vi "N-216 Contol.vi"(0 "N-216 Notifier":refnum<notifier>, 5 "Stage Action":T1={"Action"=enum."Get Position", "Axis"=[], "Setpoint"=[], "Velocity"=0.5, "Cmd Recvd?"=FALSE, "Position"=[], "Status"=enum."Error", "Misc"=variant} {"Velocity" min=0.0 max=1.0 step=0.01}, 11 "VISA In":refnum<visa-resource-name>, 13 "Axis Name":string) -> (4 "N-216 Notifier (Dup)":refnum<notifier>)   [LabVIEW 2016]
uses:
  Stages Controls/Stage Notifier Element.ctl
  Stages Controls/Stage Actions.ctl
  Stages Controls/Stage Status.ctl
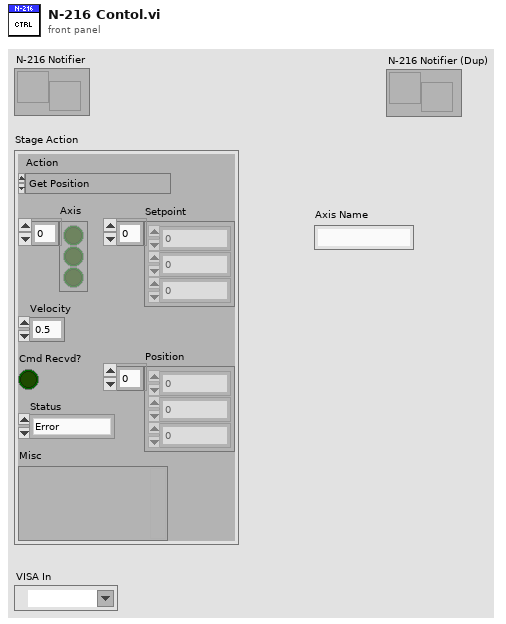
[diagram p1: front panel]
types:
  T1 = typedef "Stage Notifier Element.ctl" = cluster{"Action":T2, "Axis":bool[], "Setpoint":dbl[], "Velocity":dbl, "Cmd Recvd?":bool, "Position":dbl[], "Status":T3, "Misc":variant}
  T2 = typedef "Stage Actions.ctl" = enum16{"Get Position", "MVR", "MOVE", "HALT", "ONTARGET", "ERROR", "REFERENCE", "INIT", "VELOCITY", "STATUS", "EXIT", "HOME", "ZEROPOS", "NANOPOS", "ANALOG", "QUIT"}
  T3 = typedef "Stage Status.ctl" = enum16{"Error", "Abort", "Busy", "On Target"}
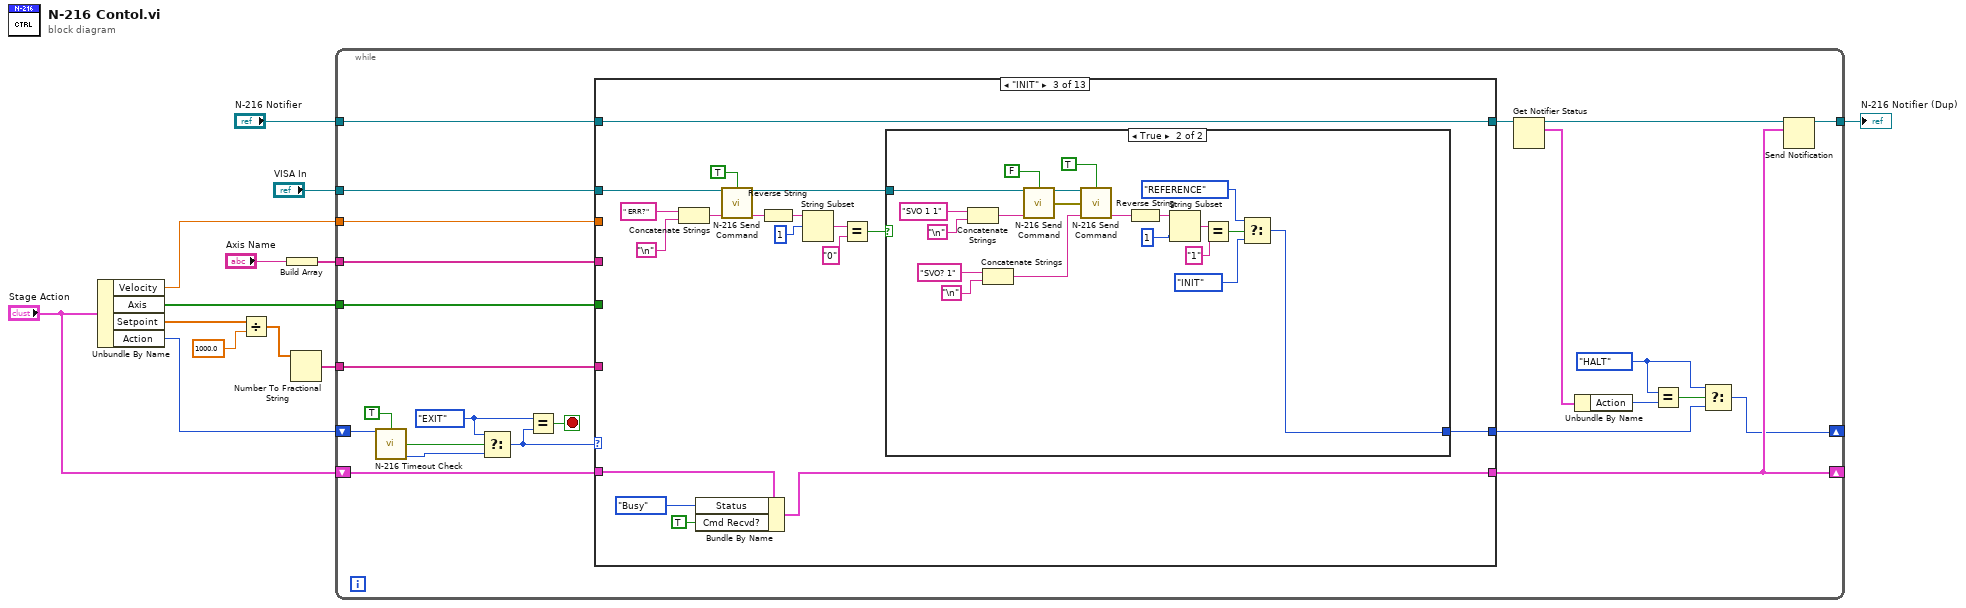
[diagram p0: block diagram]
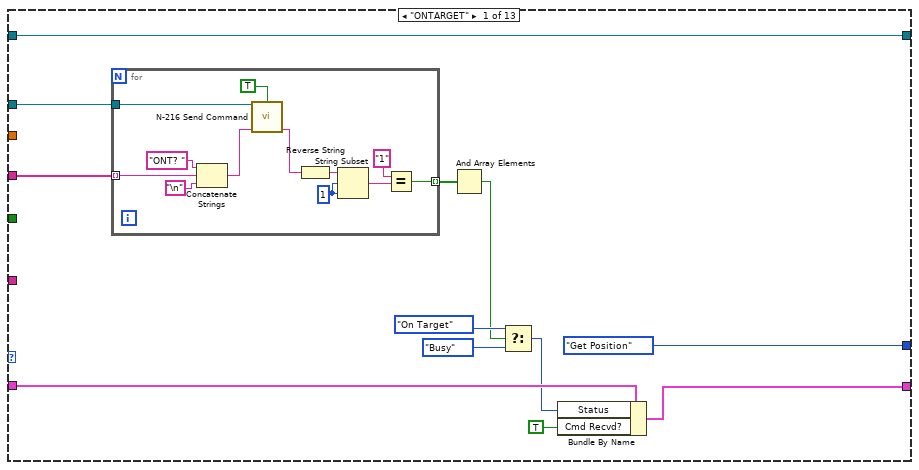
[diagram p2: hidden frame]
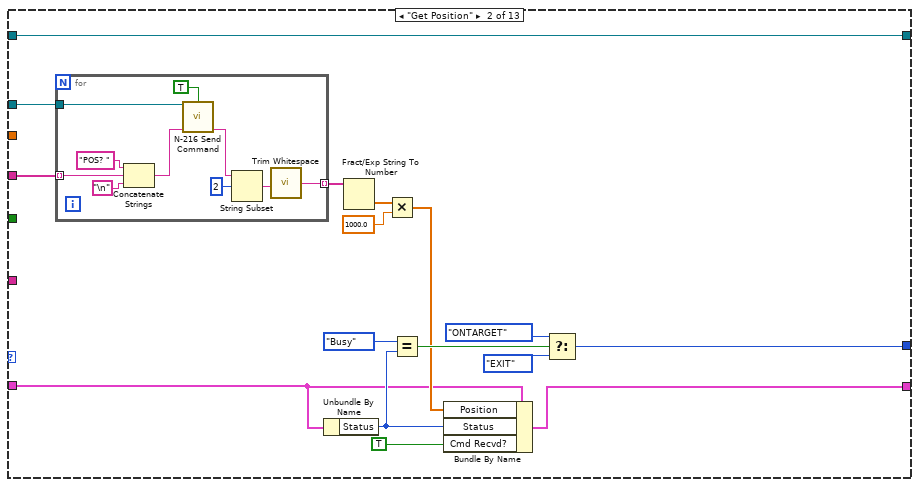
[diagram p3: hidden frame]
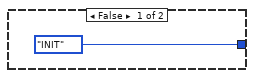
[diagram p4: hidden frame]
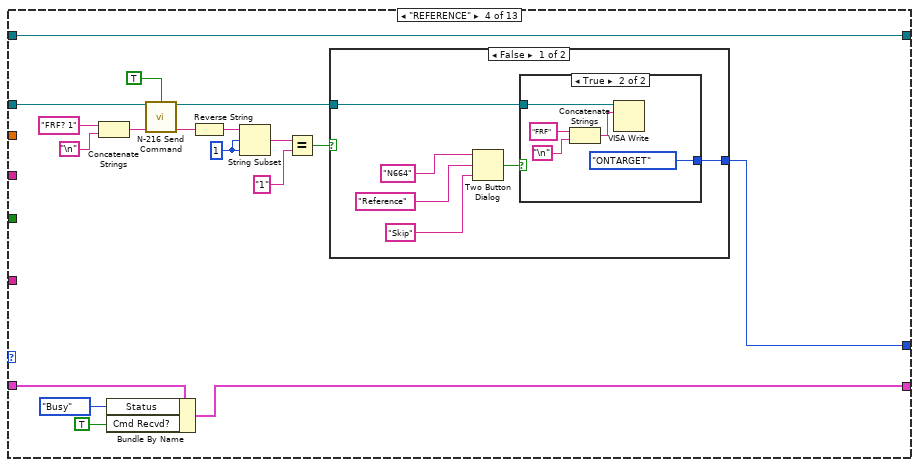
[diagram p5: hidden frame]
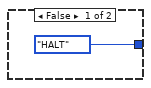
[diagram p6: hidden frame]
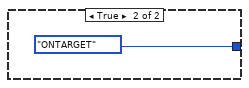
[diagram p7: hidden frame]
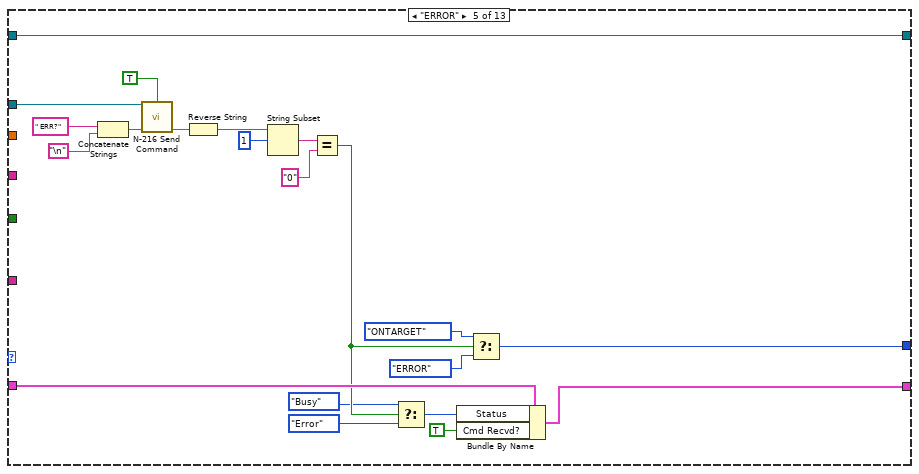
[diagram p8: hidden frame]
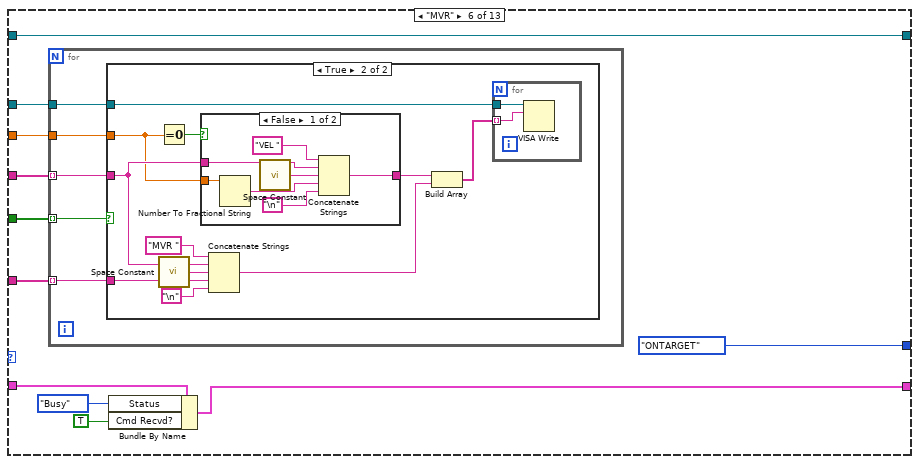
[diagram p9: hidden frame]
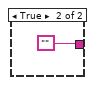
[diagram p11: hidden frame]
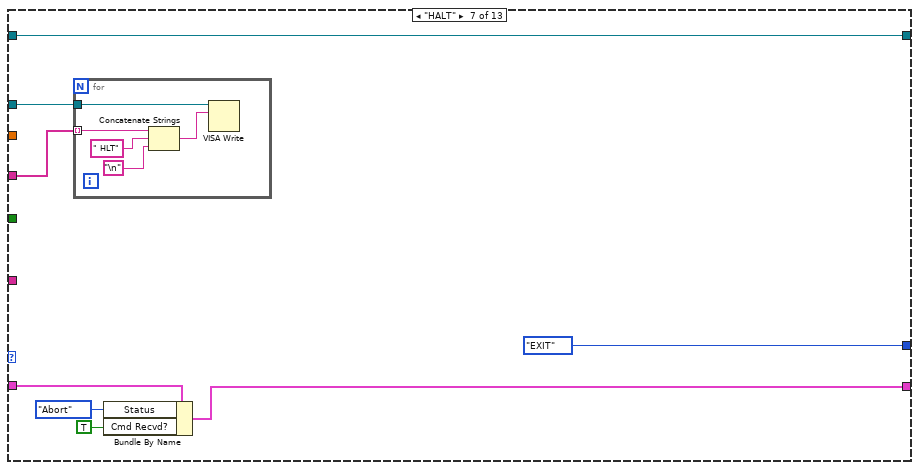
[diagram p12: hidden frame]
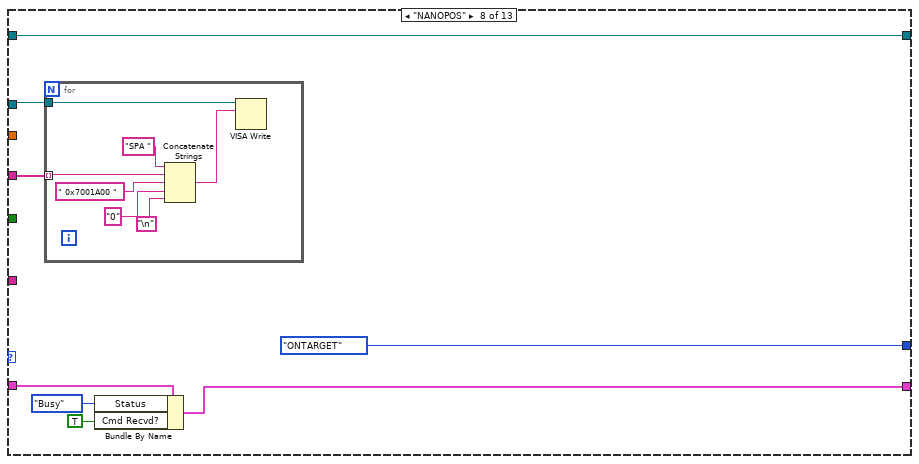
[diagram p13: hidden frame]
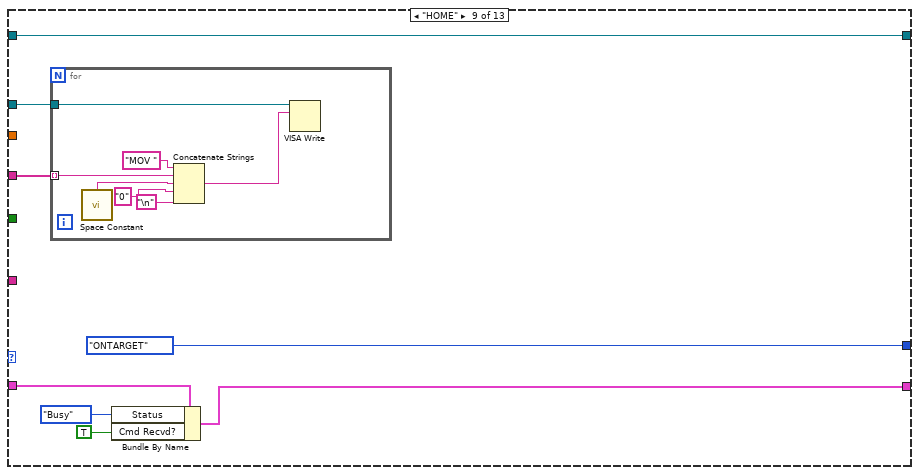
[diagram p14: hidden frame]
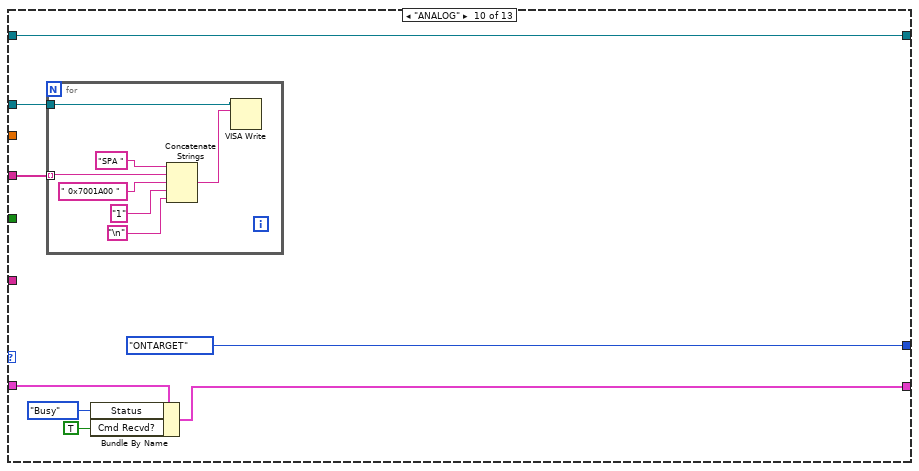
[diagram p15: hidden frame]
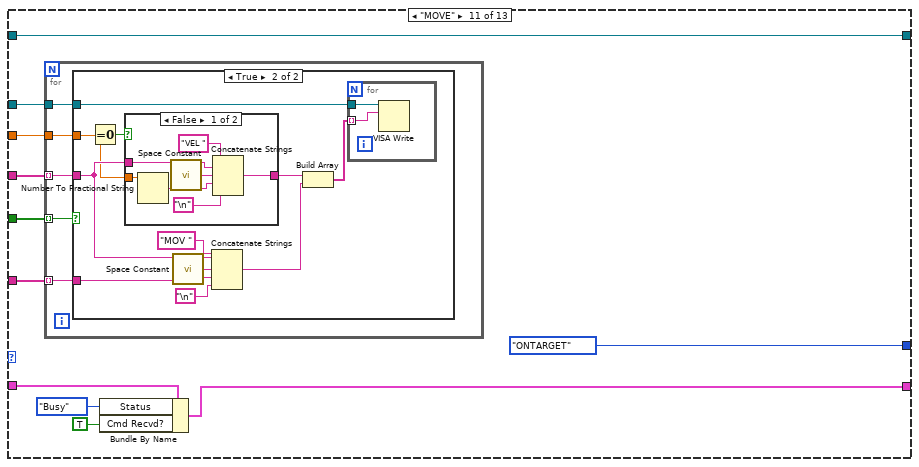
[diagram p16: hidden frame]
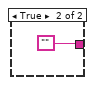
[diagram p18: hidden frame]
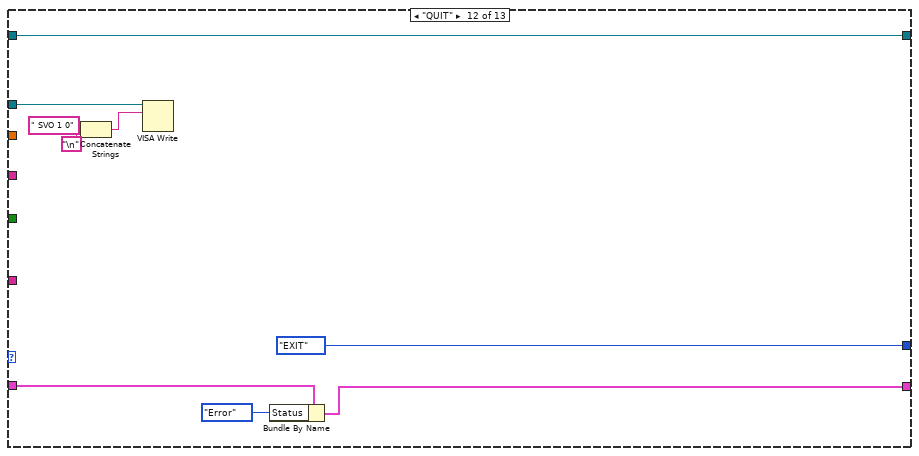
[diagram p19: hidden frame]
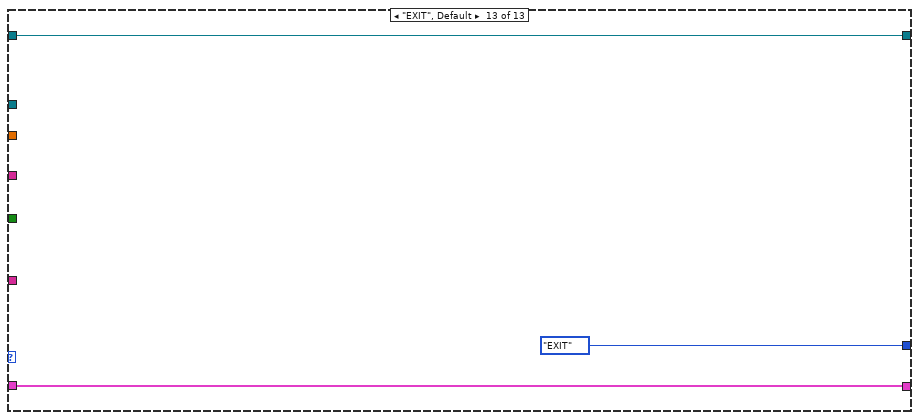
[diagram p20: hidden frame]
diagram:
  n1 = Unbundle By Name("Stage Action") -> ("Velocity"=w12:dbl, "Axis"=w11:bool[], "Setpoint"=w10:dbl[], "Action"=w9:T2)
  n2 = Divide(x=w10, y=1000.0) -> (x/y=w8:dbl[])
  n3 = Build Array("Axis Name") -> (w1:string[])
  n4 = Number To Fractional String(number=w8) -> (F-format string=w13:string[])  [unwired: 3 in]
  n5 = while {
    tunnel: w1 -> [w37]
    shift-right: [w16] -> _
    shift-left: w9 -> [w29]
    tunnel: w11 -> [w35]
    tunnel: w12 -> [w34]
    tunnel: w13 -> [w36]
    shift-right: [w31] -> _
    shift-left: "Stage Action" -> [w33]
    tunnel: "N-216 Notifier" -> [w23]
    tunnel: "VISA In" -> [w15]
    tunnel: [w14] -> w3
    stop <- w24 stop-if-true
    w19 = Stage_Actions."HALT" ("Action")
    w28 = Stage_Actions."EXIT" ("t")
    n6 = call "N-216 Timeout Check.vi"("Action"=w29, "User Input?"=TRUE) -> ("Timeout?"=w27:bool, "Action (Dup)"=w26:T2)  [unwired: 12 in]
    n7 = Select(t=w28, s=w27, f=w26) -> (s? t:f=w25:T2)
    n8 = Equal?(x=w28, y=w25) -> (x = y?=w24:bool)
    n9 = case shown="\"INIT\"" w25 {
      tunnel: w37 -> [w49 w77 _ _ _ w189 w223 w236 w251 w266 w284 _ _]
      tunnel: w15 -> [w38 w64 w93 w131 w161 w181 w217 w230 w245 w260 w274 w312 _]
      tunnel: w36 -> [_ _ _ _ _ w188 _ _ _ _ w283 _ _]
      tunnel: w35 -> [_ _ _ _ _ w187 _ _ _ _ w282 _ _]
      tunnel: w34 -> [_ _ _ _ _ w186 _ _ _ _ w281 _ _]
      tunnel: [Stage_Actions."Get Position" ("Action") w75 w105 w140 w173 Stage_Actions."ONTARGET" ("Action") Stage_Actions."EXIT" ("Action") Stage_Actions."ONTARGET" ("Action") Stage_Actions."ONTARGET" ("Action") Stage_Actions."ONTARGET" ("Action") Stage_Actions."ONTARGET" ("Action") Stage_Actions."EXIT" ("Action") Stage_Actions."EXIT" ("Action")] -> w32
      tunnel: w33 -> [w43 w62 w94 w142 w168 w183 w220 w233 w248 w263 w278 w318 w321]
      tunnel: [w39 w73 w102 w141 w170 w179 w219 w232 w247 w262 w277 w317 w321] -> w31
      tunnel: w23 -> [w40 w63 w88 w132 w163 w180 w216 w229 w244 w259 w275 w311 w320]
      tunnel: [w40 w63 w88 w132 w163 w180 w216 w229 w244 w259 w275 w311 w320] -> w18
      frame "ONTARGET" {
        n10 = for {
          tunnel: w49 -> [w61] mode=indexing
          tunnel: [w58] -> w48 mode=indexing
          tunnel: w38 -> [w53]
          w54 = 1 ("length (rest)")
          n11 = Concatenate Strings("ONT? " ("string"), w61, "\n") -> (w52:string)
          n12 = call "N-216 Send Command.vi"("VISA Ref"=w53, "Wait for Reply?"=TRUE, "Command"=w52) -> ("Response"=w51:string)  [unwired: 10 in, 2 out]
          n13 = Reverse String(1:w51) -> (0:w55:string)
          n14 = String Subset(string=w55, offset (0)=w54, length (rest)=w54) -> (substring=w60:string)
          n15 = Equal?(x="1", y=w60) -> (x = y?=w58:bool)
        }
        n16 = And Array Elements(Boolean array=w48) -> (logical AND=w44:bool)
        n17 = Select(t=Stage_Status."On Target" ("Status"), s=w44, f=Stage_Status."Busy" ("Status")) -> (s? t:f=w42:T3)
        n18 = Bundle By Name(cluster=w43, "Status"=w42, "Cmd Recvd?"=TRUE) -> (w39:T1)
      }
      frame "Get Position" {
        n19 = for {
          tunnel: w77 -> [w87] mode=indexing
          tunnel: [w86] -> w76 mode=indexing
          tunnel: w64 -> [w81]
          n20 = Concatenate Strings("POS? " ("string"), w87, "\n") -> (w79:string)
          n21 = call "N-216 Send Command.vi"("VISA Ref"=w81, "Wait for Reply?"=TRUE, "Command"=w79) -> ("Response"=w80:string)  [unwired: 10 in, 2 out]
          n22 = String Subset(string=w80, offset (0)=2) -> (substring=w82:string)  [unwired: 1 in]
          n23 = call <vilib>:"Trim Whitespace.vi"("string"=w82) -> ("trimmed string"=w86:string)  [unwired: 1 in]
        }
        n24 = Unbundle By Name(w62) -> ("Status"=w70:T3)
        n25 = Fract/Exp String To Number(string=w76) -> (number=w72:dbl[])  [unwired: 3 in, 1 out]
        n26 = Multiply(x=w72, y=1000.0) -> (x*y=w66:dbl[])
        n27 = Equal?(x=Stage_Status."Busy", y=w70) -> (x = y?=w69:bool)
        n28 = Bundle By Name(cluster=w62, "Position"=w66, "Status"=w70, "Cmd Recvd?"=TRUE) -> (w73:T1)
        n29 = Select(t=Stage_Actions."ONTARGET" ("Action"), s=w69, f=Stage_Actions."EXIT" ("Action")) -> (s? t:f=w75:T2)
      }
      frame "INIT" {
        n30 = Concatenate Strings(" ERR?" ("string"), "\n") -> (w90:string)
        n31 = Bundle By Name(cluster=w94, "Status"=Stage_Status."Busy", "Cmd Recvd?"=TRUE) -> (w102:T1)
        n32 = call "N-216 Send Command.vi"("VISA Ref"=w93, "Wait for Reply?"=TRUE, "Command"=w90) -> ("VISA Ref Out"=w92:refnum<visa-resource-name>, "Response"=w91:string)  [unwired: 10 in, 1 out]
        n33 = Reverse String(1:w91) -> (0:w98:string)
        n34 = String Subset(string=w98, offset (0)=1) -> (substring=w96:string)  [unwired: 1 in]
        n35 = Equal?(x=w96, y="0") -> (x = y?=w95:bool)
        n36 = case shown="True" w95 {
          tunnel: [Stage_Actions."INIT" ("Action") w115] -> w105
          tunnel: w92 -> [_ w114]
          frame False {
          }
          frame True {
            w124 = 1 ("length (rest)")
            n37 = Concatenate Strings("SVO 1 1" ("string"), "\n") -> (w112:string)
            n38 = Concatenate Strings("SVO? 1" ("string"), "\n") -> (w109:string)
            n39 = call "N-216 Send Command.vi"("VISA Ref"=w114, "Wait for Reply?"=FALSE, "Command"=w112) -> ("VISA Ref Out"=w110:refnum<visa-resource-name>, "Error Out"=w111:errorcluster)  [unwired: 10 in, 1 out]
            n40 = call "N-216 Send Command.vi"("VISA Ref"=w110, "Wait for Reply?"=TRUE, "Error In"=w111, "Command"=w109) -> ("Response"=w108:string)  [unwired: 9 in, 2 out]
            n41 = Reverse String(1:w108) -> (0:w123:string)
            n42 = String Subset(string=w123, offset (0)=w124, length (rest)=w124) -> (substring=w121:string)
            n43 = Equal?(x=w121, y="1") -> (x = y?=w118:bool)
            n44 = Select(t=Stage_Actions."REFERENCE" ("Action"), s=w118, f=Stage_Actions."INIT" ("Action")) -> (s? t:f=w115:T2)
          }
        }
      }
      frame "REFERENCE" {
        w134 = 1 ("length (rest)")
        n45 = Concatenate Strings("FRF? 1" ("string"), "\n") -> (w128:string)
        n46 = Bundle By Name(cluster=w142, "Status"=Stage_Status."Busy", "Cmd Recvd?"=TRUE) -> (w141:T1)
        n47 = call "N-216 Send Command.vi"("VISA Ref"=w131, "Wait for Reply?"=TRUE, "Command"=w128) -> ("VISA Ref Out"=w130:refnum<visa-resource-name>, "Response"=w129:string)  [unwired: 10 in, 1 out]
        n48 = Reverse String(1:w129) -> (0:w135:string)
        n49 = String Subset(string=w135, offset (0)=w134, length (rest)=w134) -> (substring=w137:string)
        n50 = Equal?(x=w137, y="1") -> (x = y?=w133:bool)
        n51 = case shown="False" w133 {
          tunnel: [w146 Stage_Actions."ONTARGET" ("t")] -> w140
          tunnel: w130 -> [w145 _]
          frame False {
            n52 = Two Button Dialog(message="N664", 1:"Skip" ("F button name (\"Cancel\")"), 2:"Reference" ("T button name (\"OK\")")) -> (T button?=w147:bool)
            n53 = case shown="True" w147 {
              tunnel: [Stage_Actions."HALT" ("Action") Stage_Actions."ONTARGET" ("Action")] -> w146
              tunnel: w145 -> [_ w152]
              frame False {
              }
              frame True {
                n54 = Concatenate Strings("FRF" ("string"), "\n") -> (w154:string)
                n55 = VISA Write(VISA resource name=w152, write buffer=w154) -> ()  [unwired: 1 in, 3 out]
              }
            }
          }
          frame True {
          }
        }
      }
      frame "ERROR" {
        n56 = Concatenate Strings(" ERR?" ("string"), "\n") -> (w160:string)
        n57 = call "N-216 Send Command.vi"("VISA Ref"=w161, "Wait for Reply?"=TRUE, "Command"=w160) -> ("Response"=w159:string)  [unwired: 10 in, 2 out]
        n58 = Reverse String(1:w159) -> (0:w176:string)
        n59 = String Subset(string=w176, offset (0)=1) -> (substring=w174:string)  [unwired: 1 in]
        n60 = Equal?(x=w174, y="0") -> (x = y?=w167:bool)
        n61 = Select(t=Stage_Status."Busy" ("Status"), s=w167, f=Stage_Status."Error" ("Status")) -> (s? t:f=w166:T3)
        n62 = Bundle By Name(cluster=w168, "Status"=w166, "Cmd Recvd?"=TRUE) -> (w170:T1)
        n63 = Select(t=Stage_Actions."ONTARGET" ("Action"), s=w167, f=Stage_Actions."ERROR") -> (s? t:f=w173:T2)
      }
      frame "MVR" {
        n64 = for {
          tunnel: w189 -> [w194] mode=indexing
          tunnel: w188 -> [w193] mode=indexing
          tunnel: w187 -> [w192] mode=indexing
          tunnel: w186 -> [w191]
          tunnel: w181 -> [w190]
          n65 = case shown="True" w192 {
            tunnel: w194 -> [_ w201]
            tunnel: w193 -> [_ w202]
            tunnel: w190 -> [_ w196]
            tunnel: w191 -> [_ w200]
            frame False {
            }
            frame True {
              n66 = Equal To 0?(x=w200) -> (x = 0?=w199:bool)
              n67 = call <vilib>:"Space Constant.vi"() -> ("String"=w203:string)
              n68 = case shown="False" w199 {
                tunnel: w201 -> [w211 _]
                tunnel: w200 -> [w208 _]
                tunnel: [w210 ""] -> w198
                frame False {
                  n69 = Number To Fractional String(number=w208) -> (F-format string=w209:string)  [unwired: 3 in]
                  n70 = call <vilib>:"Space Constant.vi"() -> ("String"=w214:string)
                  n71 = Concatenate Strings("VEL ", w211, w214, w209, "\n") -> (w210:string)
                }
                frame True {
                }
              }
              n72 = Concatenate Strings("MVR ", w201, w203, w202, "\n") -> (w195:string)
              n73 = Build Array(w198, w195) -> (w197:string[])
              n74 = for {
                tunnel: w197 -> [w207] mode=indexing
                tunnel: w196 -> [w206]
                n75 = VISA Write(VISA resource name=w206, write buffer=w207) -> ()  [unwired: 1 in, 3 out]
              }
            }
          }
        }
        n76 = Bundle By Name(cluster=w183, "Status"=Stage_Status."Busy", "Cmd Recvd?"=TRUE) -> (w179:T1)
      }
      frame "HALT" {
        n77 = for {
          tunnel: w223 -> [w225] mode=indexing
          tunnel: w217 -> [w224]
          n78 = Concatenate Strings(w225, " HLT" ("string"), "\n") -> (w226:string)
          n79 = VISA Write(VISA resource name=w224, write buffer=w226) -> ()  [unwired: 1 in, 3 out]
        }
        n80 = Bundle By Name(cluster=w220, "Status"=Stage_Status."Abort", "Cmd Recvd?"=TRUE) -> (w219:T1)
      }
      frame "NANOPOS" {
        n81 = for {
          tunnel: w236 -> [w240] mode=indexing
          tunnel: w230 -> [w237]
          n82 = Concatenate Strings("SPA " ("string"), w240, " 0x7001A00 " ("string"), "0", "\n") -> (w238:string)
          n83 = VISA Write(VISA resource name=w237, write buffer=w238) -> ()  [unwired: 1 in, 3 out]
        }
        n84 = Bundle By Name(cluster=w233, "Status"=Stage_Status."Busy", "Cmd Recvd?"=TRUE) -> (w232:T1)
      }
      frame "HOME" {
        n85 = for {
          tunnel: w251 -> [w254] mode=indexing
          tunnel: w245 -> [w252]
          n86 = call <vilib>:"Space Constant.vi"() -> ("String"=w255:string)
          n87 = Concatenate Strings("MOV " ("string"), w254, w255, "0" ("string"), "\n") -> (w253:string)
          n88 = VISA Write(VISA resource name=w252, write buffer=w253) -> ()  [unwired: 1 in, 3 out]
        }
        n89 = Bundle By Name(cluster=w248, "Status"=Stage_Status."Busy", "Cmd Recvd?"=TRUE) -> (w247:T1)
      }
      frame "ANALOG" {
        n90 = for {
          tunnel: w266 -> [w270] mode=indexing
          tunnel: w260 -> [w267]
          n91 = Concatenate Strings("SPA " ("string"), w270, " 0x7001A00 " ("string"), "1", "\n") -> (w269:string)
          n92 = VISA Write(VISA resource name=w267, write buffer=w269) -> ()  [unwired: 1 in, 3 out]
        }
        n93 = Bundle By Name(cluster=w263, "Status"=Stage_Status."Busy", "Cmd Recvd?"=TRUE) -> (w262:T1)
      }
      frame "MOVE" {
        n94 = for {
          tunnel: w284 -> [w289] mode=indexing
          tunnel: w283 -> [w288] mode=indexing
          tunnel: w282 -> [w287] mode=indexing
          tunnel: w281 -> [w286]
          tunnel: w274 -> [w285]
          n95 = case shown="True" w287 {
            tunnel: w289 -> [_ w296]
            tunnel: w288 -> [_ w297]
            tunnel: w285 -> [_ w290]
            tunnel: w286 -> [_ w295]
            frame False {
            }
            frame True {
              n96 = Equal To 0?(x=w295) -> (x = 0?=w294:bool)
              n97 = case shown="False" w294 {
                tunnel: w296 -> [w306 _]
                tunnel: w295 -> [w303 _]
                tunnel: [w305 ""] -> w293
                frame False {
                  n98 = Number To Fractional String(number=w303) -> (F-format string=w304:string)  [unwired: 3 in]
                  n99 = call <vilib>:"Space Constant.vi"() -> ("String"=w309:string)
                  n100 = Concatenate Strings("VEL ", w306, w309, w304, "\n") -> (w305:string)
                }
                frame True {
                }
              }
              n101 = call <vilib>:"Space Constant.vi"() -> ("String"=w298:string)
              n102 = Concatenate Strings("MOV ", w296, w298, w297, "\n") -> (w292:string)
              n103 = Build Array(w293, w292) -> (w291:string[])
              n104 = for {
                tunnel: w291 -> [w302] mode=indexing
                tunnel: w290 -> [w301]
                n105 = VISA Write(VISA resource name=w301, write buffer=w302) -> ()  [unwired: 1 in, 3 out]
              }
            }
          }
        }
        n106 = Bundle By Name(cluster=w278, "Status"=Stage_Status."Busy", "Cmd Recvd?"=TRUE) -> (w277:T1)
      }
      frame "QUIT" {
        n107 = Concatenate Strings(" SVO 1 0" ("string"), "\n") -> (w315:string)
        n108 = VISA Write(VISA resource name=w312, write buffer=w315) -> ()  [unwired: 1 in, 3 out]
        n109 = Bundle By Name(cluster=w318, "Status"=Stage_Status."Error") -> (w317:T1)
      }
      frame "EXIT", Default {
      }
    }
    n110 = Get Notifier Status(notifier=w18) -> (notifier out=w22:refnum<notifier>, current notification=w17:T1)  [unwired: 1 in, 3 out]
    n111 = Unbundle By Name(w17) -> ("Action"=w20:T2)
    n112 = Equal?(x=w19, y=w20) -> (x = y?=w21:bool)
    n113 = Select(t=w19, s=w21, f=w32) -> (s? t:f=w16:T2)
    n114 = Send Notification(notification=w31, notifier=w22) -> (notifier out=w14:refnum<notifier>)  [unwired: 1 in, 1 out]
  }
  "N-216 Notifier (Dup)" <- w3
